vi "LTC21 Check Temperature stability V1.00.vi"(5 "Address":refnum<visa-resource-name>, 6 "Use setpoint\nproximity":bool, 7 "Setpoint":dbl=0.4 format="%.3f", 8 "error in (no error)":errorcluster, 9 "Setpoint\nProximity":dbl=0.01 format="%#.3g", 10 "Seconds for\nstability":i32, 11 "Required stability":dbl=0.002 format="%#.4g") -> (0 "error out":errorcluster)   [LabVIEW 2015]
panel:
  in  "stop":bool
  out "Stability":ext=6.261161496941029e-05
  out "Waveform Chart":dbl(graph)
  out "In Range?":bool
  out "Temperature":dbl format="%.3g"
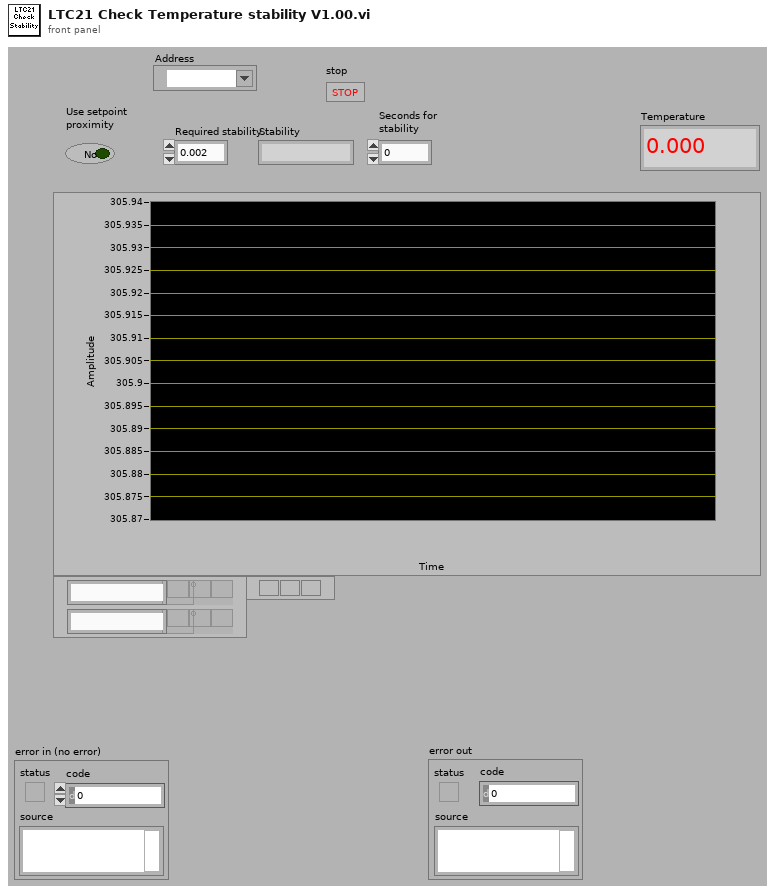
[diagram p1: front panel]
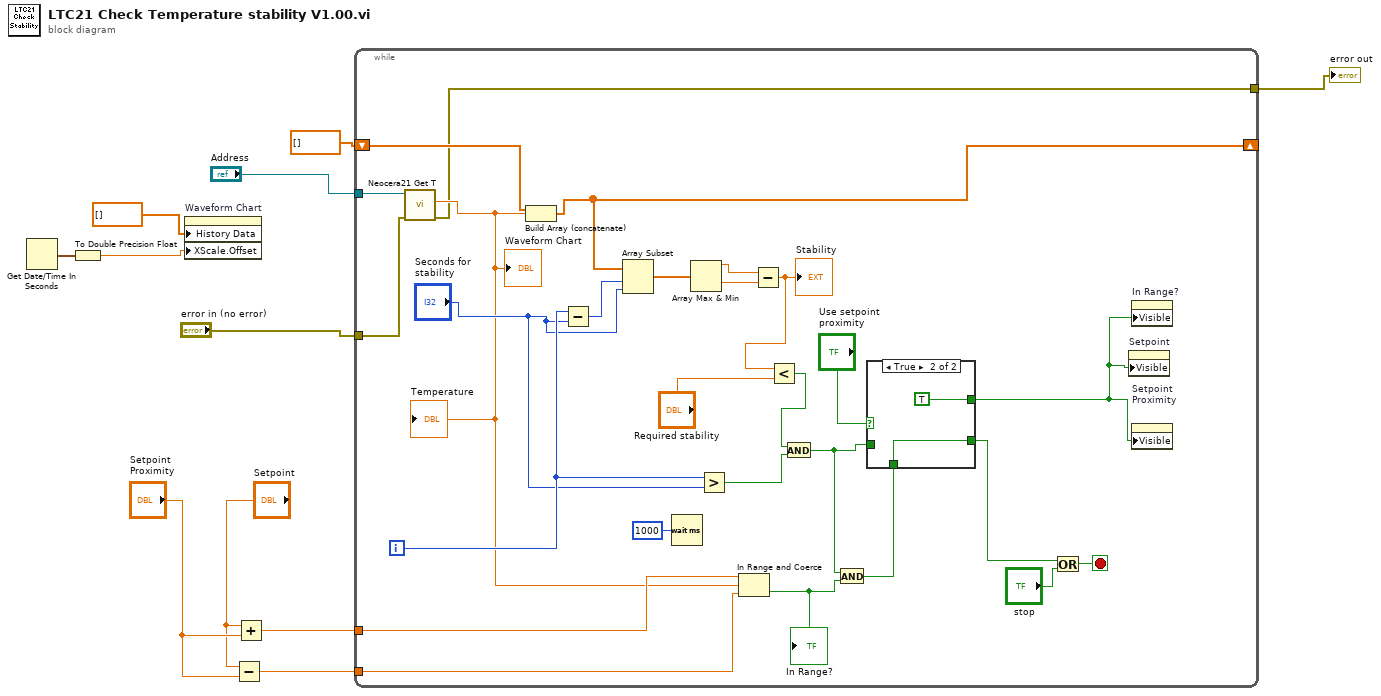
[diagram p0: block diagram]
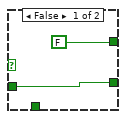
[diagram p2: hidden frame]
diagram:
  n1 = Get Date/Time In Seconds() -> (seconds since 1Jan1904=w5:timestamp)
  n2 = To Double Precision Float(number=w5) -> (double precision float=w4:dbl)
  n3 = property on="Waveform Chart" class="WFChart (strict)"("History Data"=dbl[] [], "XScale.Offset"=w4) -> ()  [unwired: 2 in, 2 out]
  n4 = Subtract(x="Setpoint", y="Setpoint\nProximity") -> (x-y=w8:dbl)
  n5 = Add(x="Setpoint", y="Setpoint\nProximity") -> (x+y=w9:dbl)
  n6 = while {
    shift-right: [w26] -> _
    shift-left: dbl[] [] -> [w28]
    tunnel: w9 -> [w24]
    tunnel: w8 -> [w23]
    tunnel: "Address" -> [w17]
    tunnel: "error in (no error)" -> [w16]
    tunnel: [w15] -> w3
    i -> [w30]
    stop <- w12 stop-if-true
    n7 = call "Neocera21 Get T.vi"("error in (no error)"=w16, "VISA Resource Name"=w17) -> ("error out"=w15:errorcluster, "Temperature"=w18:dbl)  [unwired: 6 in, 2 out]
    "Waveform Chart" <- w18
    "Temperature" <- w18
    n8 = Build Array (concatenate)(w28, w18) -> (w26:dbl[])
    n9 = Subtract(x=w30, y="Seconds for\nstability") -> (x-y=w38:i32)
    n10 = Array Subset(array=w26, index=w38, length="Seconds for\nstability") -> (w37:dbl[])
    n11 = Wait (ms)(milliseconds to wait=u32 1000) -> ()  [unwired: 1 out]
    n12 = Array Max & Min(array=w37) -> (max value=w36:dbl, min value=w35:dbl)  [unwired: 2 out]
    n13 = Greater?(x=w30, y="Seconds for\nstability") -> (0:w31:bool)
    n14 = In Range and Coerce(upper limit=w24, x=w18, lower limit=w23) -> (In Range?=w25:bool)  [unwired: 1 out]
    "In Range?" <- w25
    n15 = Subtract(x=w36, y=w35) -> (x-y=w34:dbl)
    "Stability" <- w34
    n16 = Less?(x=w34, y="Required stability") -> (x < y?=w32:bool)
    n17 = And(x=w32, y=w31) -> (x .and. y?=w21:bool)
    n18 = And(x=w21, y=w25) -> (x .and. y?=w22:bool)
    n19 = case shown="True" "Use setpoint\nproximity" {
      tunnel: [w40 w42] -> w14
      tunnel: w22 -> [_ w42]
      tunnel: w21 -> [w40 _]
      tunnel: [FALSE TRUE] -> w19
      frame False {
      }
      frame True {
      }
    }
    n20 = Or(x=w14, y="stop") -> (x .or. y?=w12:bool)
    n21 = property on="Setpoint" class="DigNum (strict)"("Visible"=w19) -> ()  [unwired: 2 in, 2 out]
    n22 = property on="In Range?" class="Bool (strict)"("Visible"=w19) -> ()  [unwired: 2 in, 2 out]
    n23 = property on="Setpoint\nProximity" class="DigNum (strict)"("Visible"=w19) -> ()  [unwired: 2 in, 2 out]
  }
  "error out" <- w3
